vi "CameraSetup.vi"(11 "Camera Setup":T1={"Format"=enum."RGB565", "size"=enum."QVGA (320x240)", "Skip frames (ms)"=2000, "autoGain"=FALSE, "autoWhitebal"=FALSE}) -> (3 "String":string)   [LabVIEW 2017]
uses:
  <userlib>/LabVIEWOpenMV/_subs/CameraSetup.ctl
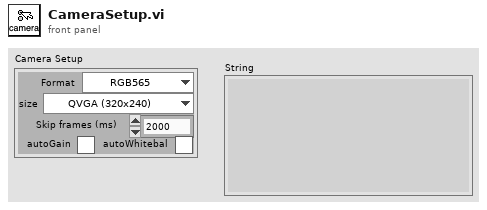
[diagram p1: front panel]
types:
  T1 = typedef "CameraSetup.ctl" = cluster{"Format":enum16{"GRAYSCALE", "RGB565", "BAYER"}, "size":enum16{"QQQQVGA (40x30)", "QQQVGA (80x60)", "QQVGA (160x120)", "QVGA (320x240)", "VGA (640x480)", "LCD (128x160)", "B64x32 (64x32)", "B64x64", "B128x64", "B128x128"}, "Skip frames (ms)":u16, "autoGain":bool, "autoWhitebal":bool}
  T2 = enum16{"QQQQVGA (40x30)", "QQQVGA (80x60)", "QQVGA (160x120)", "QVGA (320x240)", "VGA (640x480)", "LCD (128x160)", "B64x32 (64x32)", "B64x64", "B128x64", "B128x128"}
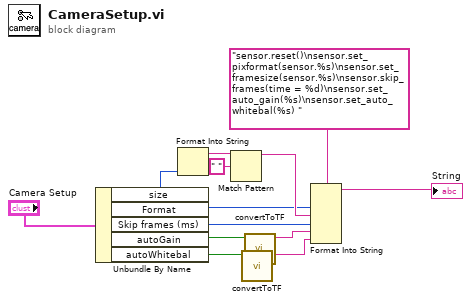
[diagram p0: block diagram]
diagram:
  n1 = Unbundle By Name("Camera Setup") -> ("size"=w9:T2, "Format"=w7:enum16{"GRAYSCALE", "RGB565", "BAYER"}, "Skip frames (ms)"=w8:u16, "autoGain"=w2:bool, "autoWhitebal"=w4:bool)
  n2 = Format Into String(w9) -> (resulting string=w10:string)  [unwired: 3 in, 1 out]
  n3 = Match Pattern(string=w10, regular expression=" ") -> (before substring=w11:string)  [unwired: 1 in, 3 out]
  n4 = call <userlib>:"convertToTF.vi"("Boolean"=w4) -> ("Text"=w3:string)  [unwired: 10 in]
  n5 = call <userlib>:"convertToTF.vi"("Boolean"=w2) -> ("Text"=w1:string)  [unwired: 10 in]
  n6 = Format Into String(format string="sensor.reset()\nsensor.set_pixformat(sensor.%s)\nsensor.set_framesize(sensor.%s)\nsensor.skip_frames(time = %d)\nsensor.set_auto_gain(%s)\nsensor.set_auto_whitebal(%s) " ("startCode"), w7, w11, w8, w1, w3) -> (resulting string=→"String":string)  [unwired: 2 in, 1 out]
